vi "Find Blood Pressure_ms.vi"(4 "Systolic Threshold":dbl, 6 "Diastolic Threshold":dbl, 8 "error in (no error)":errorcluster, 10 "Peak Amplitudes":dbl[](array[numeric]), 11 "Peak Pressures":dbl[](array[numeric])) -> (0 "error Out":errorcluster, 1 "Results":cluster{"Pressure":dbl[], "Amplitude":dbl[]}, 2 "Systolic":dbl, 3 "Diastolic":dbl)   [LabVIEW 2017]
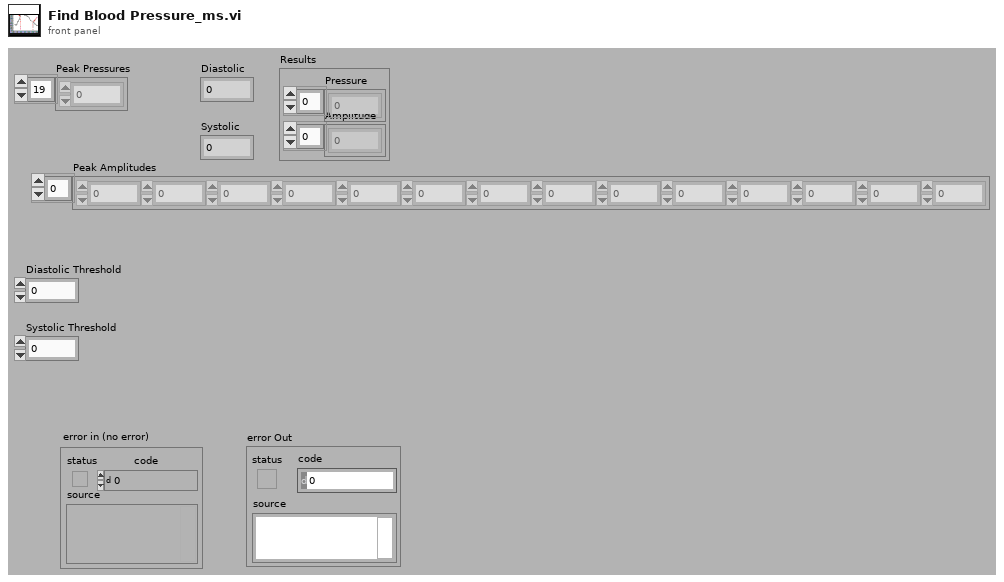
[diagram p1: front panel]
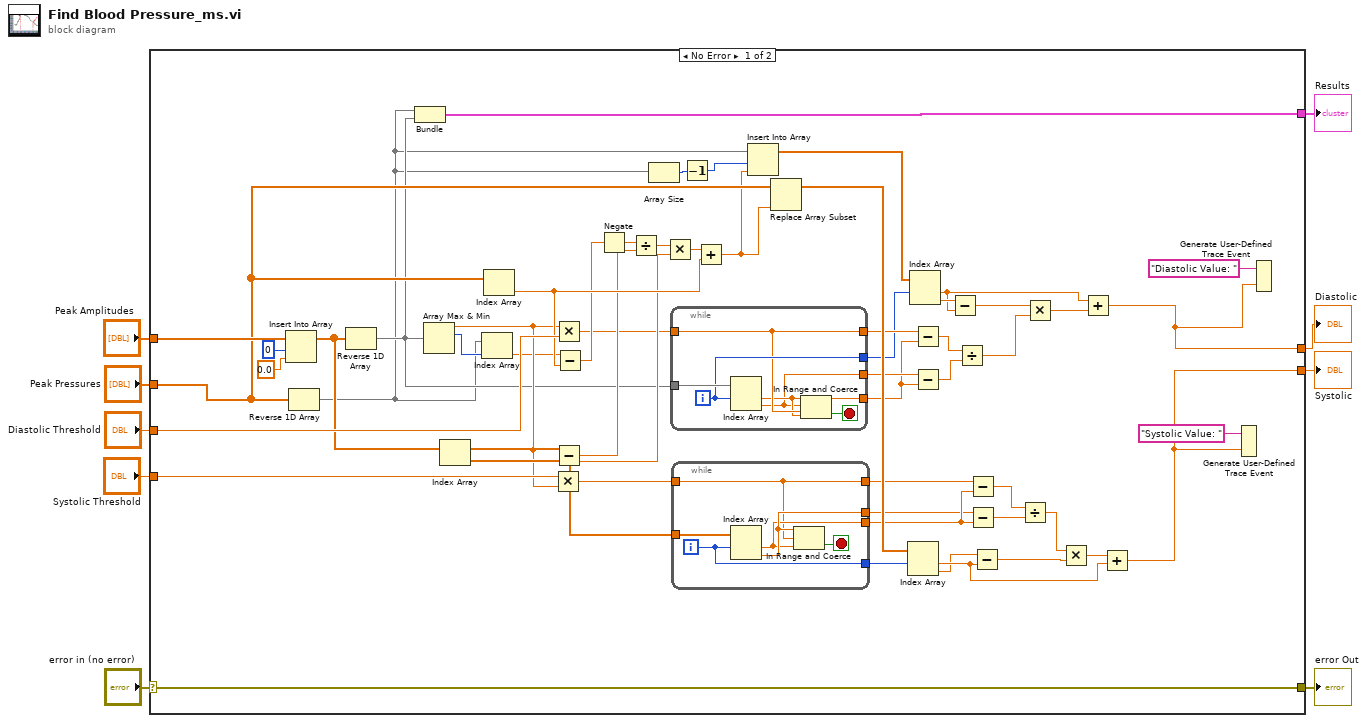
[diagram p0: block diagram]
diagram:
  n1 = case shown="No Error" "error in (no error)" {
    selector: "error in (no error)" -> [w58 w76]
    tunnel: [w13 _] -> w9
    tunnel: [w12 _] -> w8
    tunnel: "Peak Amplitudes" -> [w63 _]
    tunnel: "Peak Pressures" -> [w62 _]
    tunnel: "Diastolic Threshold" -> [w61 _]
    tunnel: "Systolic Threshold" -> [w60 _]
    tunnel: [w59 _] -> w3
    tunnel: [w58 w76] -> w1
    frame No Error {
      n2 = Insert Into Array(array=w63, index=0, new element=0.0 ("new element/subarray")) -> (w57:dbl[])
      n3 = Reverse 1D Array(array=w62) -> (reversed array=w14:dbl[])
      n4 = Reverse 1D Array(array=w57) -> (reversed array=w15:dbl[])
      n5 = Bundle(w14, w15) -> (w59:cluster{dbl[], dbl[]})  [unwired: 1 out]
      n6 = Array Max & Min(array=w15) -> (max value=w41:dbl, max index (indices)=w56:i32)  [unwired: 2 out]
      n7 = Index Array(array=w57) -> (element=w44:dbl)  [unwired: 1 in]
      n8 = Index Array(array=w14, index=w56) -> (element=w40:dbl)
      n9 = Index Array(array=w62) -> (element=w48:dbl)  [unwired: 1 in]
      n10 = Multiply(x=w60, y=w41) -> (x*y=w38:dbl)
      n11 = Multiply(x=w41, y=w61) -> (x*y=w39:dbl)
      n12 = Subtract(x=w41, y=w44) -> (x-y=w42:dbl)
      n13 = Subtract(x=w40, y=w48) -> (x-y=w45:dbl)
      n14 = Negate(x=w45) -> (-x=w46:dbl)
      n15 = Divide(x=w46, y=w42) -> (x/y=w43:dbl)
      n16 = Array Size(array=w14) -> (size(s)=w54:i32)
      n17 = Multiply(x=w43, y=w44) -> (x*y=w47:dbl)
      n18 = while {
        tunnel: w39 -> [w72]
        tunnel: w15 -> [w75]
        tunnel: [w70] -> w37
        tunnel: [w71] -> w35
        tunnel: [w72] -> w36
        tunnel: [w74] -> w32
        i -> [w74]
        stop <- w73 stop-if-true
        n19 = Index Array(array=w75, index #1=w74) -> (element #1=w71:dbl, element #2=w70:dbl)  [unwired: 1 in]
        n20 = In Range and Coerce(upper limit=w70, x=w72, lower limit=w71) -> (In Range?=w73:bool)  [unwired: 1 out]
      }
      n21 = while {
        tunnel: w38 -> [w65]
        tunnel: w57 -> [w69]
        tunnel: [w67] -> w16
        tunnel: [w66] -> w18
        tunnel: [w65] -> w17
        tunnel: [w64] -> w21
        i -> [w64]
        stop <- w68 stop-if-true
        n22 = Index Array(array=w69, index #1=w64) -> (element #1=w66:dbl, element #2=w67:dbl)  [unwired: 1 in]
        n23 = In Range and Coerce(upper limit=w67, x=w65, lower limit=w66) -> (In Range?=w68:bool)  [unwired: 1 out]
      }
      n24 = Decrement(x=w54) -> (x-1=w55:i32)
      n25 = Add(x=w47, y=w48) -> (x+y=w53:dbl)
      n26 = Insert Into Array(array=w14, index=w55, new element=w53) -> (w52:dbl[])
      n27 = Replace Array Subset(array=w62, new element=w53) -> (w51:dbl[])  [unwired: 1 in]
      n28 = Index Array(array=w51, index #1=w21) -> (element #1=w26:dbl, element #2=w22:dbl)  [unwired: 1 in]
      n29 = Index Array(array=w52, index #1=w32) -> (element #1=w27:dbl, element #2=w31:dbl)  [unwired: 1 in]
      n30 = Subtract(x=w36, y=w35) -> (x-y=w34:dbl)
      n31 = Subtract(x=w37, y=w35) -> (x-y=w33:dbl)
      n32 = Subtract(x=w31, y=w27) -> (x-y=w29:dbl)
      n33 = Divide(x=w34, y=w33) -> (x/y=w30:dbl)
      n34 = Subtract(x=w17, y=w18) -> (x-y=w19:dbl)
      n35 = Subtract(x=w16, y=w18) -> (x-y=w20:dbl)
      n36 = Subtract(x=w22, y=w26) -> (x-y=w24:dbl)
      n37 = Divide(x=w19, y=w20) -> (x/y=w23:dbl)
      n38 = Multiply(x=w29, y=w30) -> (x*y=w28:dbl)
      n39 = Multiply(x=w23, y=w24) -> (x*y=w25:dbl)
      n40 = Add(x=w27, y=w28) -> (x+y=w13:dbl)
      n41 = Add(x=w25, y=w26) -> (x+y=w12:dbl)
      n42 = Generate User-Defined Trace Event(1:w12, 2:"Systolic Value: " ("trace string")) -> ()
      n43 = Generate User-Defined Trace Event(1:w13, 2:"Diastolic Value: " ("trace string")) -> ()
    }
    frame Error {
    }
  }
  "Systolic" <- w8
  "Diastolic" <- w9
  "Results" <- w3
  "error Out" <- w1
